vi "AWG Set and Arm.vi"(7 "pulse count (0: infinite)":i32, 8 "error in (no error)":errorcluster, 9 "trigger":T1, 10 "sampling rate":T5, 11 "awg session in":T7={"type"=enum."Agilent 331xxA to 332xxA", "VISA"="", "enable 10MHz ref"=FALSE, "cmi ckd2"={"VISA"="", "clock source"=enum."Auto", "manual ref clk"=FALSE, "ref clock [Hz]"=0.0, "div mode"=enum."Set divisor directly"}, "cmi sync v3"={"VISA"="", "baud rate [bd/s]"=115200, "source"=enum."Auto", "hv range"=enum."1kV", "fsrc is fixed"=FALSE, "fsrc [Hz]"=10000000.0, "freq integ [s]"=1.0, "freq filter"=5, "trig level"=enum."TTL 5V", "chn1 mode"=enum."Source divider", "chn1 level"=enum."Positive 5V", "chn2 mode"=enum."Source divider", "chn2 level"=enum."Positive 5V", "chn2 div"=1, "chn3 mode"=enum."Chn 1 Active", "chn3 level"=enum."Positive 5V", "chn1 div entry"=enum."Calculate nearest divisor from measured fx", "chn1 dev limit [%]"=1.0, "chn1 check dev"=FALSE}, "trigger"={"source"=enum."Immediate", "level [V]"=0.0, "coupling"=enum."DC", "slope"=enum."POS"}, "HMF2500 cfg"={"Baud Rate"=9600, "Parity"=0, "Data Bits"=8, "Flow Control"=4}} {"HMF2500 cfg"."Flow Control" items=["None", "XON/XOFF", "RTS/CTS", "XON/XOFF & RTS/CTS", "DTR/DSR", "XON/XOFF & DTR/DSR"]; "HMF2500 cfg"."Data Bits" items=["7"=7, "8"=8]; "HMF2500 cfg"."Parity" items=["None", "Odd", "Even", "Mark", "Space"]; "HMF2500 cfg"."Baud Rate" items=["300"=300, "600"=600, "1200"=1200, "2400"=2400, "4800"=4800, "9600"=9600, "19200"=19200]; "cmi sync v3"."chn2 div" min=1 max=100000000 step=1; "cmi sync v3"."fsrc [Hz]" format="%_8p"}) -> (0 "error out":errorcluster, 3 "awg session out":T7={"type"=enum."Agilent 331xxA to 332xxA", "VISA"="", "enable 10MHz ref"=FALSE, "cmi ckd2"={"VISA"="", "clock source"=enum."Auto", "manual ref clk"=FALSE, "ref clock [Hz]"=0.0, "div mode"=enum."Set divisor directly"}, "cmi sync v3"={"VISA"="", "baud rate [bd/s]"=115200, "source"=enum."Auto", "hv range"=enum."1kV", "fsrc is fixed"=FALSE, "fsrc [Hz]"=10000000.0, "freq integ [s]"=1.0, "freq filter"=5, "trig level"=enum."TTL 5V", "chn1 mode"=enum."Source divider", "chn1 level"=enum."Positive 5V", "chn2 mode"=enum."Source divider", "chn2 level"=enum."Positive 5V", "chn2 div"=1, "chn3 mode"=enum."Chn 1 Active", "chn3 level"=enum."Positive 5V", "chn1 div entry"=enum."Calculate nearest divisor from measured fx", "chn1 dev limit [%]"=1.0, "chn1 check dev"=FALSE}, "trigger"={"source"=enum."Immediate", "level [V]"=0.0, "coupling"=enum."DC", "slope"=enum."POS"}, "HMF2500 cfg"={"Baud Rate"=9600, "Parity"=0, "Data Bits"=8, "Flow Control"=4}} {"HMF2500 cfg"."Flow Control" items=["None", "XON/XOFF", "RTS/CTS", "XON/XOFF & RTS/CTS", "DTR/DSR", "XON/XOFF & DTR/DSR"]; "HMF2500 cfg"."Data Bits" items=["7"=7, "8"=8]; "HMF2500 cfg"."Parity" items=["None", "Odd", "Even", "Mark", "Space"]; "HMF2500 cfg"."Baud Rate" items=["300"=300, "600"=600, "1200"=1200, "2400"=2400, "4800"=4800, "9600"=9600, "19200"=19200]; "cmi sync v3"."chn2 div" min=1 max=100000000 step=1; "cmi sync v3"."fsrc [Hz]" format="%_8p"})   [LabVIEW 2020, in "AWG.lvlib"]
doc: "AWG wrapper: This sets the AWG to desired frequency and arms it. No pulses are generated here. Waiting for trigger!"
uses:
  AWG.lvlib
  AWG Session.ctl
  AWG Type.ctl
  CMI Clock Divider v2/CMI ckd2 Session.ctl
  CMI Clock Divider v2/CMI ckd2 Source Mode.ctl
  CMI Clock Divider v2/CMI ckd2 Divisor Mode.ctl
  CMI Sync V3/CMI Sync V3 session.ctl
  CMI Sync V3/Configure/CMI Sync V3 Reference Clock Source.ctl
  CMI Sync V3/Configure/CMI Sync V3 HV input Range.ctl
  CMI Sync V3/Configure/CMI Sync V3 Trigger Input Level.ctl
  CMI Sync V3/Configure/CMI Sync V3 Channel 1 Mode.ctl
  CMI Sync V3/Configure/CMI Sync V3 Channel Output Levels.ctl
  CMI Sync V3/Configure/CMI Sync V3 Channel 2 Mode.ctl
  CMI Sync V3/Configure/CMI Sync V3 Channel 3 Mode.ctl
  CMI Sync V3/Configure/CMI Sync V3 Channel 1 Divisor Entry Mode.ctl
  externals needed for AWG/ADC Trig Config.ctl
  externals needed for AWG/ADC Trig Mode Source.ctl
  externals needed for AWG/ADC Trig Coupling.ctl
  externals needed for AWG/ADC Trig Slope.ctl
  RaS HMF2500/HMF2500 Config.ctl
  externals needed for AWG/3458A Sampling Rate.ctl
  AWG Clock Setup Mode.ctl
  Agilent 33XXX Series/Agilent 33XXX Series.lvlib
  AFG3000/Tektronix AFG 3000 Series.lvlib
  CMI Sync V3/CMI Sync Unit V3.lvlib
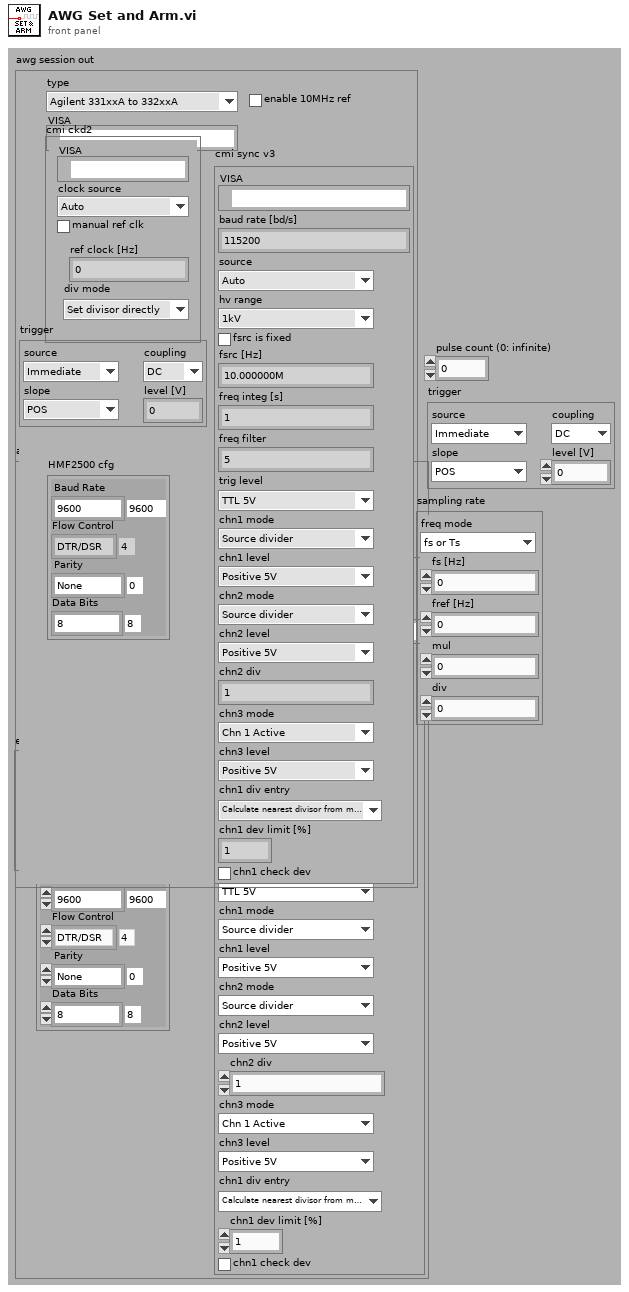
[diagram p1: front panel]
types:
  T1 = typedef "ADC Trig Config.ctl" = cluster{"source":T2, "level [V]":dbl, "coupling":T3, "slope":T4}
  T2 = typedef "ADC Trig Mode Source.ctl" = enum16{"Immediate", "External", "Level"}
  T3 = typedef "ADC Trig Coupling.ctl" = enum16{"DC", "AC"}
  T4 = typedef "ADC Trig Slope.ctl" = enum16{"POS", "NEG"}
  T5 = typedef "3458A Sampling Rate.ctl" = cluster{"freq mode":T6, "fs [Hz]":dbl, "fref [Hz]":dbl, "mul":dbl, "div":dbl}
  T6 = typedef "AWG.lvlib/AWG Clock Setup Mode.ctl" = enum16{"fs or Ts", "fs or Ts with fref", "fref/N", "fref*M/N", "fref*Ratio"}
  T7 = typedef "AWG.lvlib/AWG Session.ctl" = cluster{"type":T8, "VISA":refnum<visa-resource-name>, "enable 10MHz ref":bool, "cmi ckd2":T9, "cmi sync v3":T12, "trigger":T1, "HMF2500 cfg":T21}
  T8 = typedef "AWG.lvlib/AWG Type.ctl" = enum16{"Agilent 331xxA to 332xxA", "Agilent 335xxA to 336xxA", "Tektronix AFG3101C", "R&S HMF25xx", "CMI Clock Divider v2", "CMI Sync Unit V3", "dummy"}
  T9 = typedef "AWG.lvlib/CMI ckd2 Session.ctl" = cluster{"VISA":refnum<visa-resource-name>, "clock source":T10, "manual ref clk":bool, "ref clock [Hz]":dbl, "div mode":T11}
  T10 = typedef "AWG.lvlib/CMI ckd2 Source Mode.ctl" = enum16{"Auto", "LF clock", "HF clock", "Internal"}
  T11 = typedef "AWG.lvlib/CMI ckd2 Divisor Mode.ctl" = enum16{"Set divisor directly", "Set divisor by frequency"}
  T12 = typedef "AWG.lvlib/CMI Sync Unit V3.lvlib/CMI Sync V3 session.ctl" = cluster{"VISA":refnum<visa-resource-name>, "baud rate [bd/s]":i32, "source":T13, "hv range":T14, "fsrc is fixed":bool, "fsrc [Hz]":dbl, "freq integ [s]":dbl, "freq filter":i32, "trig level":T15, "chn1 mode":T16, "chn1 level":T17, "chn2 mode":T18, "chn2 level":T17, "chn2 div":i32, "chn3 mode":T19, "chn3 level":T17, "chn1 div entry":T20, "chn1 dev limit [%]":dbl, "chn1 check dev":bool}
  T13 = typedef "AWG.lvlib/CMI Sync Unit V3.lvlib/CMI Sync V3 Reference Clock Source.ctl" = enum16{"Auto", "Internal", "Logic", "Sine", "HV"}
  T14 = typedef "AWG.lvlib/CMI Sync Unit V3.lvlib/CMI Sync V3 HV input Range.ctl" = enum16{"10V", "60V", "250V", "1kV"}
  T15 = typedef "AWG.lvlib/CMI Sync Unit V3.lvlib/CMI Sync V3 Trigger Input Level.ctl" = enum16{"LVCMOS 3V3", "TTL 5V"}
  T16 = typedef "AWG.lvlib/CMI Sync Unit V3.lvlib/CMI Sync V3 Channel 1 Mode.ctl" = enum16{"Source divider", "DDS absolute", "DDS ratio", "DDS ratio M/N"}
  T17 = typedef "AWG.lvlib/CMI Sync Unit V3.lvlib/CMI Sync V3 Channel Output Levels.ctl" = enum16{"Positive 3V3", "Negative 3V3", "Positive 5V", "Negative 5V"}
  T18 = typedef "AWG.lvlib/CMI Sync Unit V3.lvlib/CMI Sync V3 Channel 2 Mode.ctl" = enum16{"Source divider", "Chn 1 divide"}
  T19 = typedef "AWG.lvlib/CMI Sync Unit V3.lvlib/CMI Sync V3 Channel 3 Mode.ctl" = enum16{"Chn 1 Active", "Chn 2 Active", "Chn 1 Trigger", "Chn 2 Trigger", "Gate", "PPS", "10MHz"}
  T20 = typedef "AWG.lvlib/CMI Sync Unit V3.lvlib/CMI Sync V3 Channel 1 Divisor Entry Mode.ctl" = enum16{"Set divisor directly", "Calculate nearest divisor from measured fx"}
  T21 = typedef "AWG.lvlib/HMF2500 Config.ctl" = cluster{"Baud Rate":u32, "Parity":u16, "Data Bits":u16, "Flow Control":u16}
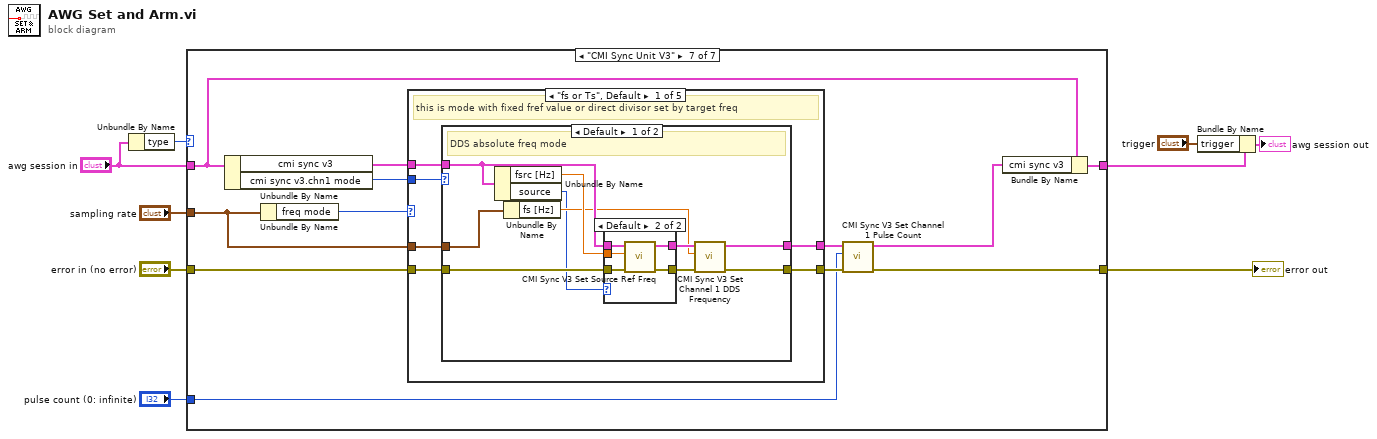
[diagram p0: block diagram]
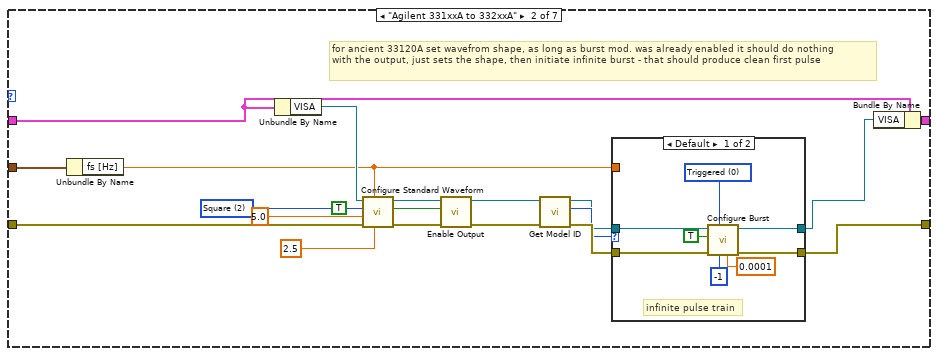
[diagram p3: hidden frame]
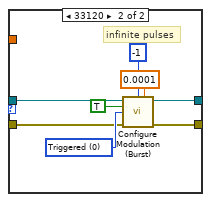
[diagram p4: hidden frame]
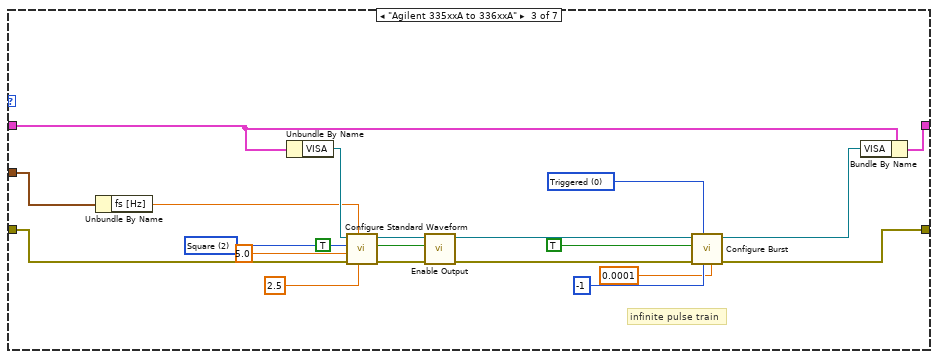
[diagram p5: hidden frame]
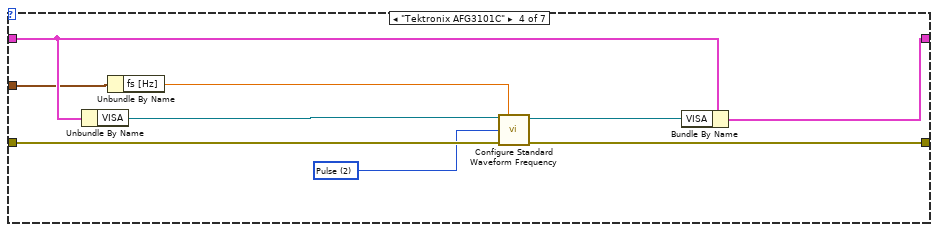
[diagram p6: hidden frame]
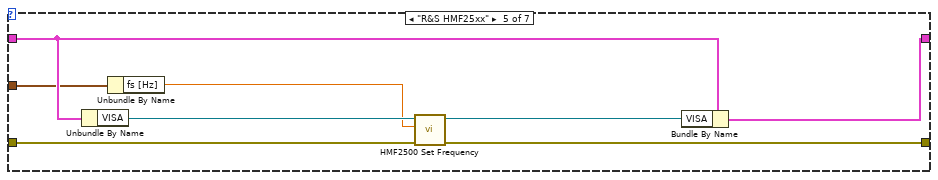
[diagram p7: hidden frame]
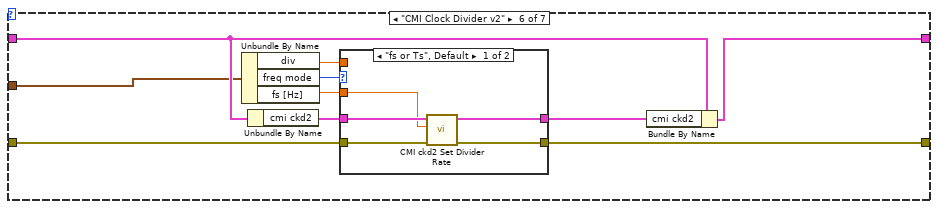
[diagram p8: hidden frame]
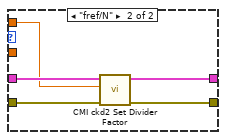
[diagram p9: hidden frame]
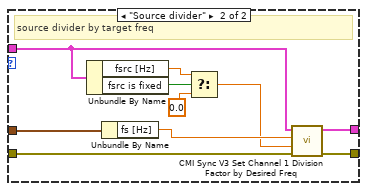
[diagram p11: hidden frame]
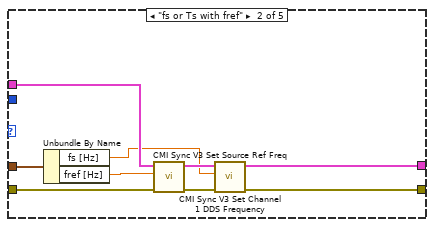
[diagram p12: hidden frame]
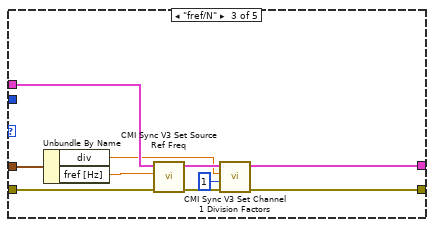
[diagram p13: hidden frame]
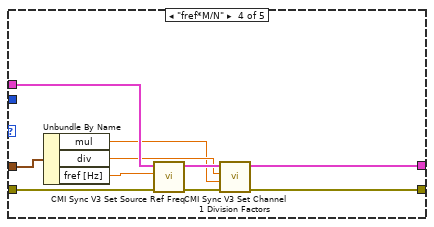
[diagram p14: hidden frame]
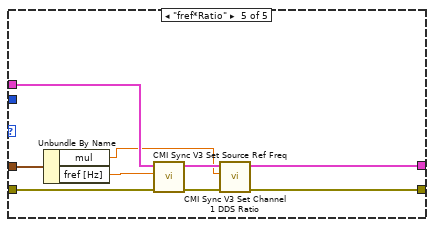
[diagram p15: hidden frame]
diagram:
  n1 = Unbundle By Name("awg session in") -> ("type"=w9:T8)
  n2 = case shown="\"CMI Sync Unit V3\"" w9 {
    tunnel: "error in (no error)" -> [w11 w25 w56 w72 w80 w93 w114]
    tunnel: [w11 w14 w49 w69 w78 w88 w108] -> w7
    tunnel: "awg session in" -> [w10 w29 w66 w75 w83 w91 w110]
    tunnel: [w10 w30 w65 w74 w82 w87 w111] -> w4
    tunnel: "sampling rate" -> [_ w15 w57 w68 w77 w89 w112]
    tunnel: "pulse count (0: infinite)" -> [_ _ _ _ _ _ w107]
    frame Default {
    }
    frame "Agilent 331xxA to 332xxA" {
      w28 = u16 2 items=["DC", "Sine", "Square", "Triangle", "Ramp", "Pulse", "Noise", "Sinc", "Negative Ramp", "Exponential Rise", "Exponential Fall", "Cardiac"] ("Waveform Function (1: Sine)")
      # "for ancient 33120A set wavefrom shape, as long as burst mod. was already enabled it should do nothing\nwith the output, just sets the shape, then initiate infinite burst - that should produce clean first pulse"
      n3 = Unbundle By Name(w15) -> ("fs [Hz]"=w12:dbl)
      n4 = Unbundle By Name(w29) -> ("VISA"=w26:refnum<visa-resource-name>)
      n5 = call "Configure Standard Waveform.vi"("DC Offset (0.00 V)"=2.5, "Frequency (1000 Hz)"=w12, "error in (no error)"=w25, "Amplitude (1)"=5.0, "Waveform Function (1: Sine)"=w28, "VISA resource name"=w26) -> ("error out"=w23:errorcluster, "VISA resource name out"=w22:refnum<visa-resource-name>)  [unwired: 4 in]
      n6 = call "Enable Output.vi"("error in (no error)"=w23, "Enable Output  (T: Enable)"=TRUE, "VISA resource name"=w22) -> ("error out"=w20:errorcluster, "VISA resource name out"=w19:refnum<visa-resource-name>)  [unwired: 7 in]
      n7 = call "Get Model ID.vi"("error in (no error)"=w20, "VISA resource name"=w19) -> ("error out"=w18:errorcluster, "model ID"=w17:u32, "VISA resource name out"=w16:refnum<visa-resource-name>)  [unwired: 7 in]
      n8 = case shown="Default" w17 {
        tunnel: [w37 w43] -> w14
        tunnel: [w36 w42] -> w13
        tunnel: w12 -> [_ _]
        tunnel: w18 -> [w38 w41]
        tunnel: w16 -> [w35 w40]
        frame Default {
          w34 = u16 0 items=["Triggered", "Gated"] ("Burst Mode (0: Triggered)")
          # "infinite pulse train"
          n9 = call "Configure Burst.vi"("Burst Period (1 s)"=0.0001, "Burst Count (1)"=-1, "Burst Mode (0: Triggered)"=w34, "error in (no error)"=w38, "Enable Burst (T: Enable)"=TRUE, "VISA resource name"=w35) -> ("error out"=w37:errorcluster, "VISA resource name out"=w36:refnum<visa-resource-name>)  [unwired: 4 in]
        }
        frame 33120 {
          w44 = u16 0 items=["Triggered", "Gated"] ("Burst Modulation Mode (0: Triggered)")
          # "infinite pulses"
          n10 = call "Configure Modulation (Burst).vi"("VISA resource name"=w40, "Burst Count (1)"=-1, "Burst Period (1 s)"=0.0001, "Enable Burst Modulation (T: Enable)"=TRUE, "Burst Modulation Mode (0: Triggered)"=w44, "error in (no error)"=w41) -> ("VISA resource name out"=w42:refnum<visa-resource-name>, "error out"=w43:errorcluster)  [unwired: 8 in]
        }
      }
      n11 = Bundle By Name(cluster=w29, "VISA"=w13) -> (w30:T7)
    }
    frame "Agilent 335xxA to 336xxA" {
      w55 = u16 0 items=["Triggered", "Gated"] ("Burst Mode (0: Triggered)")
      w64 = u16 2 items=["DC", "Sine", "Square", "Triangle", "Ramp", "Pulse", "Noise", "Sinc", "Negative Ramp", "Exponential Rise", "Exponential Fall", "Cardiac"] ("Waveform Function (1: Sine)")
      # "infinite pulse train"
      n12 = Unbundle By Name(w57) -> ("fs [Hz]"=w47:dbl)
      n13 = Unbundle By Name(w66) -> ("VISA"=w58:refnum<visa-resource-name>)
      n14 = call "Configure Standard Waveform.vi"("DC Offset (0.00 V)"=2.5, "Frequency (1000 Hz)"=w47, "error in (no error)"=w56, "Amplitude (1)"=5.0, "Waveform Function (1: Sine)"=w64, "VISA resource name"=w58) -> ("error out"=w61:errorcluster, "VISA resource name out"=w60:refnum<visa-resource-name>)  [unwired: 4 in]
      n15 = call "Enable Output.vi"("error in (no error)"=w61, "Enable Output  (T: Enable)"=TRUE, "VISA resource name"=w60) -> ("error out"=w51:errorcluster, "VISA resource name out"=w50:refnum<visa-resource-name>)  [unwired: 7 in]
      n16 = call "Configure Burst.vi"("Burst Period (1 s)"=0.0001, "Burst Count (1)"=-1, "Burst Mode (0: Triggered)"=w55, "error in (no error)"=w51, "Enable Burst (T: Enable)"=TRUE, "VISA resource name"=w50) -> ("error out"=w49:errorcluster, "VISA resource name out"=w48:refnum<visa-resource-name>)  [unwired: 4 in]
      n17 = Bundle By Name(cluster=w66, "VISA"=w48) -> (w65:T7)
    }
    frame "Tektronix AFG3101C" {
      w71 = u16 2 items=["Sine", "Square", "Pulse", "Ramp", "Noise", "DC", "Sin(x)/x", "Gaussian", "Lorentz", "Exponential Rise", "Exponential Decay", "Haversine"] ("Waveform Function (0: Sine)")
      n18 = Unbundle By Name(w75) -> ("VISA"=w73:refnum<visa-resource-name>)
      n19 = Unbundle By Name(w68) -> ("fs [Hz]"=w67:dbl)
      n20 = call "Configure Standard Waveform Frequency.vi"("VISA resource name"=w73, "Frequency (1000 Hz)"=w67, "Waveform Function (0: Sine)"=w71, "error in (no error)"=w72) -> ("VISA resource name out"=w70:refnum<visa-resource-name>, "error out"=w69:errorcluster)  [unwired: 10 in]
      n21 = Bundle By Name(cluster=w75, "VISA"=w70) -> (w74:T7)
    }
    frame "R&S HMF25xx" {
      n22 = Unbundle By Name(w83) -> ("VISA"=w81:refnum<visa-resource-name>)
      n23 = Unbundle By Name(w77) -> ("fs [Hz]"=w76:dbl)
      n24 = call "HMF2500 Set Frequency.vi"("error in (no error)"=w80, "frequency [Hz] (1000)"=w76, "VISA in"=w81) -> ("error out"=w78:errorcluster, "VISA out"=w79:refnum<visa-resource-name>)  [unwired: 7 in]
      n25 = Bundle By Name(cluster=w83, "VISA"=w79) -> (w82:T7)
    }
    frame "CMI Clock Divider v2" {
      n26 = Unbundle By Name(w89) -> ("div"=w84:dbl, "freq mode"=w85:T6, "fs [Hz]"=w86:dbl)
      n27 = Unbundle By Name(w91) -> ("cmi ckd2"=w92:T9)
      n28 = case shown="\"fs or Ts\", Default" w85 {
        tunnel: w93 -> [w98 w103]
        tunnel: w92 -> [w96 w100]
        tunnel: [w94 w101] -> w90
        tunnel: [w97 w102] -> w88
        tunnel: w86 -> [w95 _]
        tunnel: w84 -> [_ w99]
        frame "fs or Ts", Default {
          n29 = call "CMI ckd2 Set Divider Rate.vi"("error in"=w98, "clock rate [Hz]"=w95, "session"=w96) -> ("error out"=w97:errorcluster, "session out"=w94:T9)  [unwired: 5 in, 2 out]
        }
        frame "fref/N" {
          n30 = call "CMI ckd2 Set Divider Factor.vi"("error in"=w103, "division factor (1)"=w99, "session"=w100) -> ("error out"=w102:errorcluster, "session out"=w101:T9)  [unwired: 7 in]
        }
      }
      n31 = Bundle By Name(cluster=w91, "cmi ckd2"=w90) -> (w87:T7)
    }
    frame "CMI Sync Unit V3" {
      n32 = Unbundle By Name(w110) -> ("cmi sync v3"=w113:T12, "cmi sync v3.chn1 mode"=w104:T16)
      n33 = Unbundle By Name(w112) -> ("freq mode"=w115:T6)
      n34 = case shown="\"fs or Ts\", Default" w115 {
        tunnel: w114 -> [w121 w157 w167 w177 w186]
        tunnel: w113 -> [w117 w156 w166 w176 w185]
        tunnel: w112 -> [w120 w154 w164 w174 w183]
        tunnel: [w119 w151 w161 w171 w180] -> w109
        tunnel: [w118 w150 w160 w170 w179] -> w106
        tunnel: w104 -> [w116 _ _ _ _]
        frame "fs or Ts", Default {
          # "this is mode with fixed fref value or direct divisor set by target freq"
          n35 = case shown="Default" w116 {
            tunnel: w121 -> [w131 w148]
            tunnel: w120 -> [w129 w147]
            tunnel: [w127 w145] -> w119
            tunnel: [w126 w144] -> w118
            tunnel: w117 -> [w125 w143]
            frame Default {
              # "DDS absolute freq mode"
              n36 = Unbundle By Name(w125) -> ("fsrc [Hz]"=w124:dbl, "source"=w122:T13)
              n37 = Unbundle By Name(w129) -> ("fs [Hz]"=w123:dbl)
              n38 = case shown="Default" w122 {
                tunnel: w131 -> [w133 w138]
                tunnel: [w133 w137] -> w130
                tunnel: [w132 w136] -> w128
                tunnel: w125 -> [w132 w135]
                tunnel: w124 -> [_ w134]
                frame "Internal" {
                }
                frame Default {
                  n39 = call "CMI Sync V3 Set Source Ref Freq.vi"("error in"=w138, "Expected reference frequency [Hz]"=w134, "session in"=w135) -> ("error out"=w137:errorcluster, "session out"=w136:T12)  [unwired: 7 in]
                }
              }
              n40 = call "CMI Sync V3 Set Channel 1 DDS Frequency.vi"("error in"=w130, "DDS absolute [Hz] (1 MHz)"=w123, "session in"=w128) -> ("error out"=w127:errorcluster, "session out"=w126:T12)  [unwired: 7 in]
            }
            frame "Source divider" {
              # "source divider by target freq"
              n41 = Unbundle By Name(w143) -> ("fsrc [Hz]"=w141:dbl, "fsrc is fixed"=w142:bool)
              n42 = Unbundle By Name(w147) -> ("fs [Hz]"=w146:dbl)
              n43 = Select(t=w141, s=w142, f=0.0) -> (s? t:f=w139:dbl)
              n44 = call "CMI Sync V3 Set Channel 1 Division Factor by Desired Freq.vi"("error in"=w148, "explicit ref freq [Hz] (0: auto estimate)"=w139, "target output freq [Hz]"=w146, "session in"=w143) -> ("error out"=w145:errorcluster, "session out"=w144:T12)  [unwired: 4 in, 2 out]
            }
          }
        }
        frame "fs or Ts with fref" {
          n45 = Unbundle By Name(w154) -> ("fs [Hz]"=w149:dbl, "fref [Hz]"=w153:dbl)
          n46 = call "CMI Sync V3 Set Source Ref Freq.vi"("error in"=w157, "Expected reference frequency [Hz]"=w153, "session in"=w156) -> ("error out"=w155:errorcluster, "session out"=w152:T12)  [unwired: 7 in]
          n47 = call "CMI Sync V3 Set Channel 1 DDS Frequency.vi"("error in"=w155, "DDS absolute [Hz] (1 MHz)"=w149, "session in"=w152) -> ("error out"=w151:errorcluster, "session out"=w150:T12)  [unwired: 7 in]
        }
        frame "fref/N" {
          n48 = Unbundle By Name(w164) -> ("div"=w159:dbl, "fref [Hz]"=w163:dbl)
          n49 = call "CMI Sync V3 Set Source Ref Freq.vi"("error in"=w167, "Expected reference frequency [Hz]"=w163, "session in"=w166) -> ("error out"=w165:errorcluster, "session out"=w162:T12)  [unwired: 7 in]
          n50 = call "CMI Sync V3 Set Channel 1 Division Factors.vi"("error in"=w165, "DDS multiplier (1)"=1, "Divider (10)"=w159, "session in"=w162) -> ("error out"=w161:errorcluster, "session out"=w160:T12)  [unwired: 6 in]
        }
        frame "fref*M/N" {
          n51 = Unbundle By Name(w174) -> ("mul"=w168:dbl, "div"=w169:dbl, "fref [Hz]"=w173:dbl)
          n52 = call "CMI Sync V3 Set Source Ref Freq.vi"("error in"=w177, "Expected reference frequency [Hz]"=w173, "session in"=w176) -> ("error out"=w175:errorcluster, "session out"=w172:T12)  [unwired: 7 in]
          n53 = call "CMI Sync V3 Set Channel 1 Division Factors.vi"("error in"=w175, "DDS multiplier (1)"=w168, "Divider (10)"=w169, "session in"=w172) -> ("error out"=w171:errorcluster, "session out"=w170:T12)  [unwired: 6 in]
        }
        frame "fref*Ratio" {
          n54 = Unbundle By Name(w183) -> ("mul"=w178:dbl, "fref [Hz]"=w182:dbl)
          n55 = call "CMI Sync V3 Set Source Ref Freq.vi"("error in"=w186, "Expected reference frequency [Hz]"=w182, "session in"=w185) -> ("error out"=w184:errorcluster, "session out"=w181:T12)  [unwired: 7 in]
          n56 = call "CMI Sync V3 Set Channel 1 DDS Ratio.vi"("error in"=w184, "DDS ratio (1.0)"=w178, "session in"=w181) -> ("error out"=w180:errorcluster, "session out"=w179:T12)  [unwired: 7 in]
        }
      }
      n57 = call "CMI Sync V3 Set Channel 1 Pulse Count.vi"("error in"=w109, "Pulse count (0: infinite)"=w107, "session in"=w106) -> ("error out"=w108:errorcluster, "session out"=w105:T12)  [unwired: 7 in]
      n58 = Bundle By Name(cluster=w110, "cmi sync v3"=w105) -> (w111:T7)
    }
  }
  "error out" <- w7
  n59 = Bundle By Name(cluster=w4, "trigger"="trigger") -> (→"awg session out":T7)
